vi "Trumpf_RD_DataBaseUpload_AutoReport.vi"(2 "error in (no error)":errorcluster, 3 "Bar_LIV_Data":path=path "D:/LabVIEW_prog/Trumpf_Database_Connect/TestData/Averaging_DM17-20_Post.xlsx") -> (0 "error out":errorcluster)   [LabVIEW 2017]
doc: "This example allows you to perform several tasks on the specified table in a database named LabVIEW.mdb located in the LabVIEW examples>>database directory.\n\nThis VI is running when you open it. Select one of the tabs and enter the appropriate data. Press the Go button to complete the displayed tab option.\n\nAutomatic - This option inserts a new record into the specified table. The record is specified by a cluster containing the correct number of elements and of the data types defined by the specified table. \n\nSQL Query - This option performs the specified SQL query.\n\nParameterized SQL Query - This option performs the specified SQL query as a parameterized SQL Query. This method is faster and more efficient than directly executing an SQL query because it sets up all the parameters prior to doing the command."
uses:
  <vilib>/addons/database/Connection.llb/DB Tools Open Connec (String).vi
  <vilib>/addons/database/NI_Database_API.lvlib
panel:
  out "Written Bar LIV Data":T1(array[cluster])
  out "Database Column":string[](array[string])
  # "Overview: Demonstrates how to insert records into databases, and perform SQL queries.\nRequirements: Database Connectivity Toolkit\nInstructions:\nRun the VI."
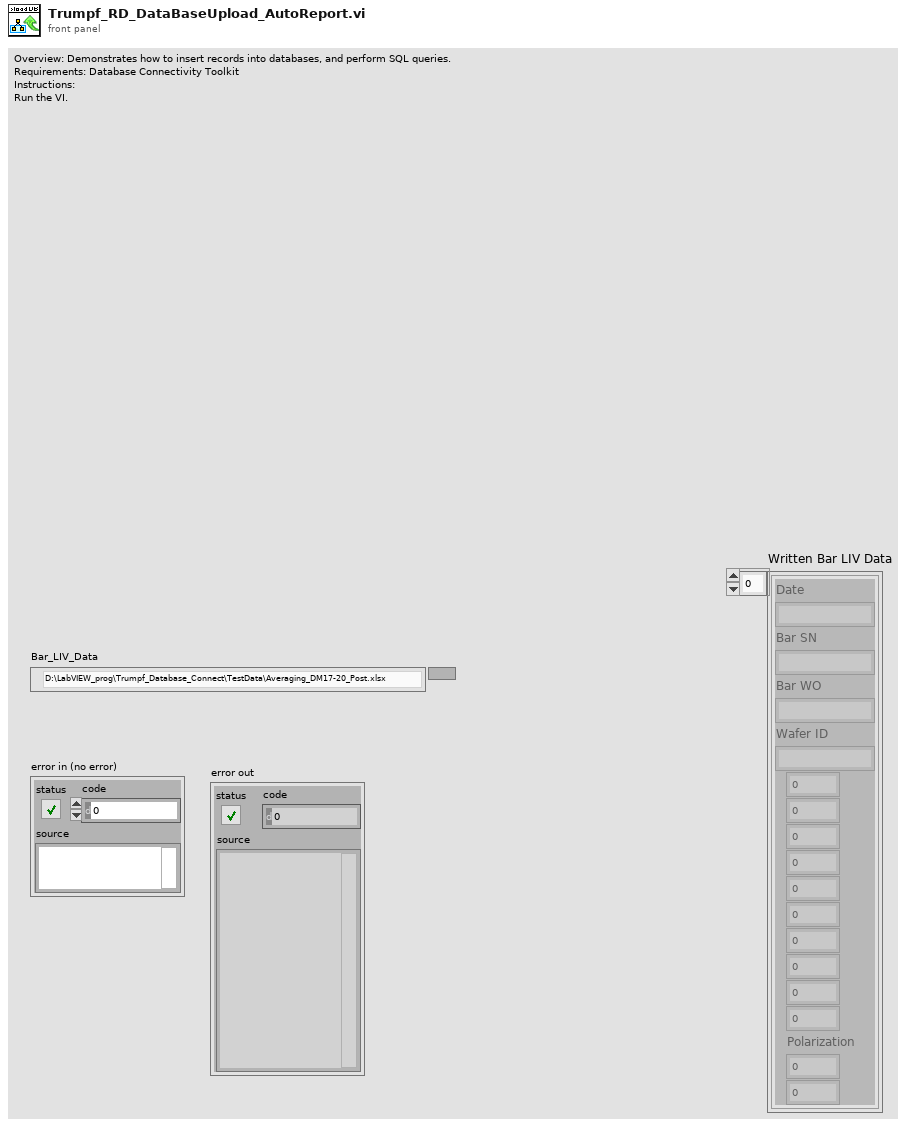
[diagram p1: front panel]
types:
  T1 = cluster{"Date":string, "Bar SN":string, "Bar WO":string, "Wafer ID":string, dbl, dbl, dbl, dbl, dbl, dbl, dbl, dbl, dbl, dbl, "Polarization":dbl, dbl}[]
  T2 = cluster{"Date":string, "LIV Data":dbl[][], "Polarization":dbl, "Bar SN":string, "Bar WO":string, "Wafer ID":string}
  T3 = typedef "NI_Database_API.lvlib/Conn ObjectReference.ctl" = refnum<k1>
  T4 = cluster{"Date":string, "Bar SN":string, "Bar WO":string, "Wafer ID":string, dbl, dbl, dbl, dbl, dbl, dbl, dbl, dbl, dbl, dbl, "Polarization":dbl, dbl}
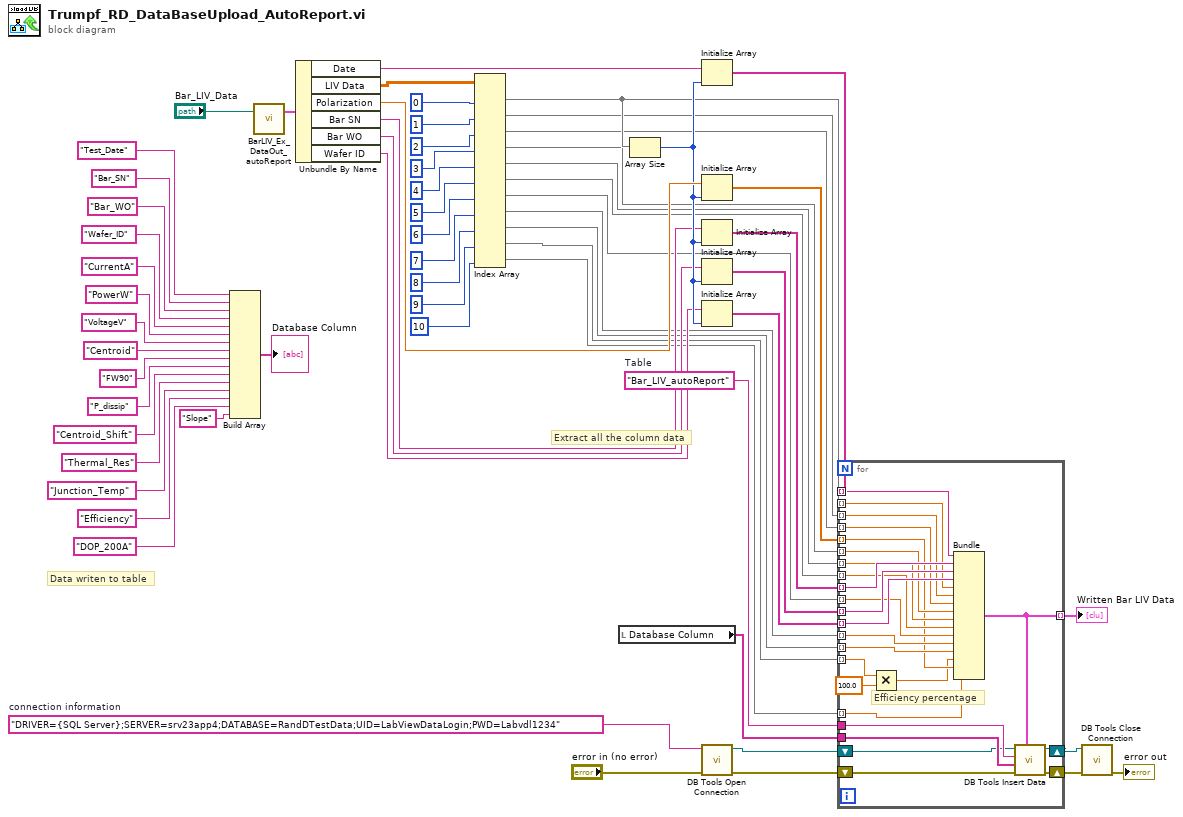
[diagram p0: block diagram]
diagram:
  w8 = "Bar_LIV_autoReport"  # Table
  w58 = "DRIVER={SQL Server};SERVER=srv23app4;DATABASE=RandDTestData;UID=LabViewDataLogin;PWD=Labvdl1234"  # connection information
  # "Data writen to table"
  # "Extract all the column data"
  n1 = Build Array("Test_Date", "Bar_SN", "Bar_WO", "Wafer_ID", "CurrentA", "PowerW", "VoltageV", "Centroid", "FW90", "P_dissip", "Centroid_Shift", "Thermal_Res", "Junction_Temp", "Efficiency", "DOP_200A", "Slope") -> (→"Database Column":string[])
  n2 = call "BarLIV_Ex_DataOut_autoReport.vi"("Bar_LIV_AutoRep"="Bar_LIV_Data") -> ("BarLIV AutoRep Output"=w54:T2)  [unwired: 1 in, 1 out]
  n3 = Unbundle By Name(w54) -> ("Date"=w27:string, "LIV Data"=w41:dbl[][], "Polarization"=w29:dbl, "Bar SN"=w26:string, "Bar WO"=w25:string, "Wafer ID"=w24:string)
  n4 = Index Array(array=w41, index (col) #1=0 ("disabled index (col)"), index (col) #2=1 ("index (col)"), index (col) #3=2 ("index (col)"), index (col) #4=3 ("index (col)"), index (col) #5=4 ("index (col)"), index (col) #6=5 ("index (col)"), index (col) #7=6 ("index (col)"), index (col) #8=7 ("index (col)"), index (col) #9=8 ("index (col)"), index (col) #10=9 ("index (col)"), index (col) #11=10 ("index (col)")) -> (element #1=w19:dbl[], element #2=w17:dbl[], element #3=w18:dbl[], element #4=w16:dbl[], element #5=w15:dbl[], element #6=w14:dbl[], element #7=w13:dbl[], element #8=w12:dbl[], element #9=w11:dbl[], element #10=w1:dbl[], element #11=w10:dbl[])  [unwired: 11 in]
  n5 = local read "Database Column"() -> (w7:string[])
  n6 = Array Size(array=w19) -> (size(s)=w28:i32)
  n7 = Initialize Array(w27, w28) -> (w23:string[])
  n8 = Initialize Array(w29, w28) -> (w9:dbl[])
  n9 = Initialize Array(w26, w28) -> (w22:string[])
  n10 = Initialize Array(w25, w28) -> (w21:string[])
  n11 = Initialize Array(w24, w28) -> (w20:string[])
  n12 = call-poly <vilib>:"DB Tools Open Connection.vi"("error in (no error)"="error in (no error)", "connection information"=w58) -> ("error out"=w6:errorcluster, "connection reference"=w4:T3)  [unwired: 6 in]
  n13 = for {
    tunnel: w23 -> [w88] mode=indexing
    tunnel: w22 -> [w87] mode=indexing
    tunnel: w21 -> [w86] mode=indexing
    tunnel: w20 -> [w85] mode=indexing
    tunnel: w19 -> [w84] mode=indexing
    tunnel: w18 -> [w82] mode=indexing
    tunnel: w17 -> [w83] mode=indexing
    tunnel: w16 -> [w81] mode=indexing
    tunnel: w15 -> [w80] mode=indexing
    tunnel: w14 -> [w79] mode=indexing
    tunnel: w13 -> [w78] mode=indexing
    tunnel: w12 -> [w77] mode=indexing
    tunnel: w11 -> [w76] mode=indexing
    tunnel: w1 -> [w66] mode=indexing
    tunnel: w9 -> [w75] mode=indexing
    tunnel: w10 -> [w74] mode=indexing
    tunnel: w8 -> [w73]
    tunnel: w7 -> [w72]
    shift-right: [w70] -> w5
    shift-left: w6 -> [w71]
    shift-right: [w69] -> w3
    shift-left: w4 -> [w68]
    tunnel: [w67] -> w2 mode=indexing
    # "Efficiency percentage"
    n14 = Multiply(x=w66, y=100.0) -> (x*y=w65:dbl)
    n15 = Bundle("Date"=w88, "Bar SN"=w87, "Bar WO"=w86, "Wafer ID"=w85, w84, w83, w82, w81, w80, w79, w78, w77, w76, w65, "Polarization"=w75, w74) -> (w67:T4)  [unwired: 1 in]
    n16 = call <vilib>:"DB Tools Insert Data.vi"("data"=w67, "error in (no error)"=w71, "columns"=w72, "table"=w73, "connection reference"=w68) -> ("error out"=w70:errorcluster, "connection reference out"=w69:T3)  [unwired: 5 in]
  }
  "Written Bar LIV Data" <- w2
  n17 = call <vilib>:"DB Tools Close Connection.vi"("error in (no error)"=w5, "connection reference"=w3) -> ("error out"=→"error out":errorcluster)  [unwired: 5 in]
